vi "dfd_Cascaded SOS Form I Normalization.vi"(7 "scale type":T1, 9 "coefficients b":dbl[](array[numeric]) format="%.2f", 10 "coefficients a":dbl[](array[numeric]) format="%.2f", 11 "x":dbl[](array[numeric])) -> (2 "norm":dbl[](array[numeric]) format="%.2f", 3 "y":dbl[](array[numeric]))   [LabVIEW 2017, in "NI_DigFilter_FXP.lvlib"]
uses:
  <vilib>/addons/Digital Filter Design/NI_DigFilter_FXP.lvlib
  <vilib>/addons/Digital Filter Design/_Objects.llb/DFD Coef Norm Type.ctl
  <vilib>/addons/Digital Filter Design/NI_DigFilterLicensed.lvlib
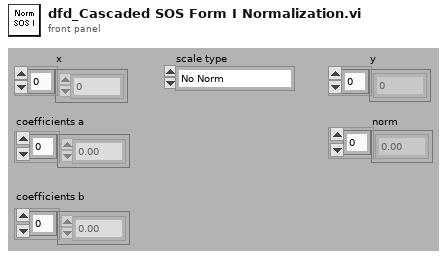
[diagram p1: front panel]
types:
  T1 = typedef "NI_DigFilterLicensed.lvlib/DFD Coef Norm Type.ctl" = enum16{"No Norm", "Time Domain 1-Norm", "Time Domain 2-Norm", "Time Domain Inf-Norm"}
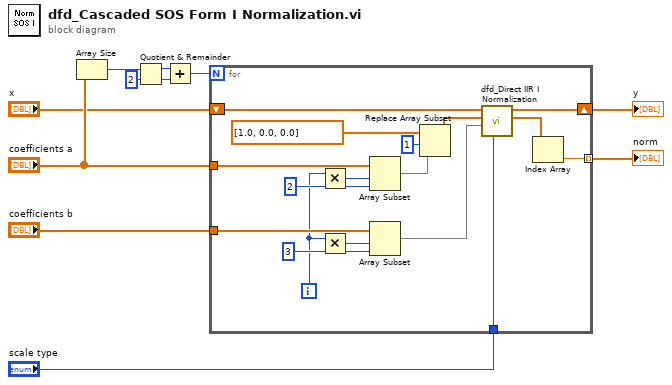
[diagram p0: block diagram]
diagram:
  n1 = Array Size(array="coefficients a") -> (size(s)=w6:i32)
  n2 = Quotient & Remainder(x=w6, y=2) -> (x-y*floor(x/y)=w10:i32, floor(x/y)=w9:i32)
  n3 = Add(x=w10, y=w9) -> (x+y=w5:i32)
  n4 = for {
    N: w5 -> [_]
    tunnel: "coefficients b" -> [w28]
    tunnel: "coefficients a" -> [w27]
    shift-right: [w15] -> w3
    shift-left: "x" -> [w21]
    tunnel: [w12] -> w1 mode=indexing
    tunnel: "scale type" -> [w14]
    i -> [w22]
    w24 = 2
    w26 = 3
    n5 = Multiply(x=w22, y=w24) -> (x*y=w23:i32)
    n6 = Multiply(x=w22, y=w26) -> (x*y=w25:i32)
    n7 = Array Subset(array=w27, index=w23, length=w24) -> (w18:dbl[])
    n8 = Array Subset(array=w28, index=w25, length=w26) -> (w20:dbl[])
    n9 = Replace Array Subset(array=dbl[] [1.0, 0.0, 0.0], new element=w18, index=1) -> (w16:dbl[])
    n10 = call <vilib>:"dfd_Direct IIR I Normalization.vi"("scale type"=w14, "coefficients b"=w20, "coefficients a"=w16, "x"=w21) -> ("norm"=w13:dbl[], "y"=w15:dbl[])  [unwired: 6 out]
    n11 = Index Array(array=w13) -> (element=w12:dbl)  [unwired: 1 in]
  }
  "norm" <- w1
  "y" <- w3
